vi "Set Trigger Mode.vi"(11 "mode":u32) -> ()   [LabVIEW 2021, in "vmmso.lvlib"]
doc: "DLL_API void WINAPI SetTriggerMode(unsigned int mode);"
uses:
  vmmso.lvlib
  vmmso.dll
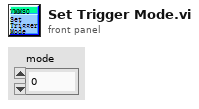
[diagram p1: front panel]
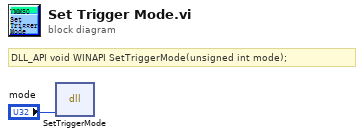
[diagram p0: block diagram]
diagram:
  # "DLL_API void WINAPI SetTriggerMode(unsigned int mode);"
  n1 = dll-call lib="D:/labviewdemo/LabviewDemo 21/vmmso/vmmso.*" fn="SetTriggerMode"("mode"="mode") -> ()  [unwired: 5 in, 2 out]
